vi "WLAN_FrameAnalysis.vi"(8 "error in (no error)":errorcluster, 10 "Decode SC":bool, 11 "input cluster":cluster{"t0":dbl, "dt":dbl, "Y":cdb[]}) -> (0 "error out":errorcluster, 1 "Constellation":cdb[](graph), 2 "Modulation parameter":T1, 3 "output bits":i8[](array[numeric]), 4 "Frequency offset":dbl, 5 "SIG valid?":bool, 6 "FFT":dbl[](graph))   [LabVIEW 2022 SP3]
panel:
  out "x+y":dbl
  out "Frequency offset(LTF)":dbl
  out "Frequency offset corrected signal 2":cluster{"t0":dbl, "dt":dbl, "Y":dbl[]}(graph)
  out "size(s) 3":i32
  out "size(s) 2":i32
  out "size(s)":i32
  out "Symbol numbers":i32
  out "encoded bit numbers":u32
  out "original bit numbers":u32
  out "Channel Esitimate":dbl[](graph)
  out "Frequency offset corrected signal":cluster{"t0":dbl, "dt":dbl, "Y":dbl[]}(graph)
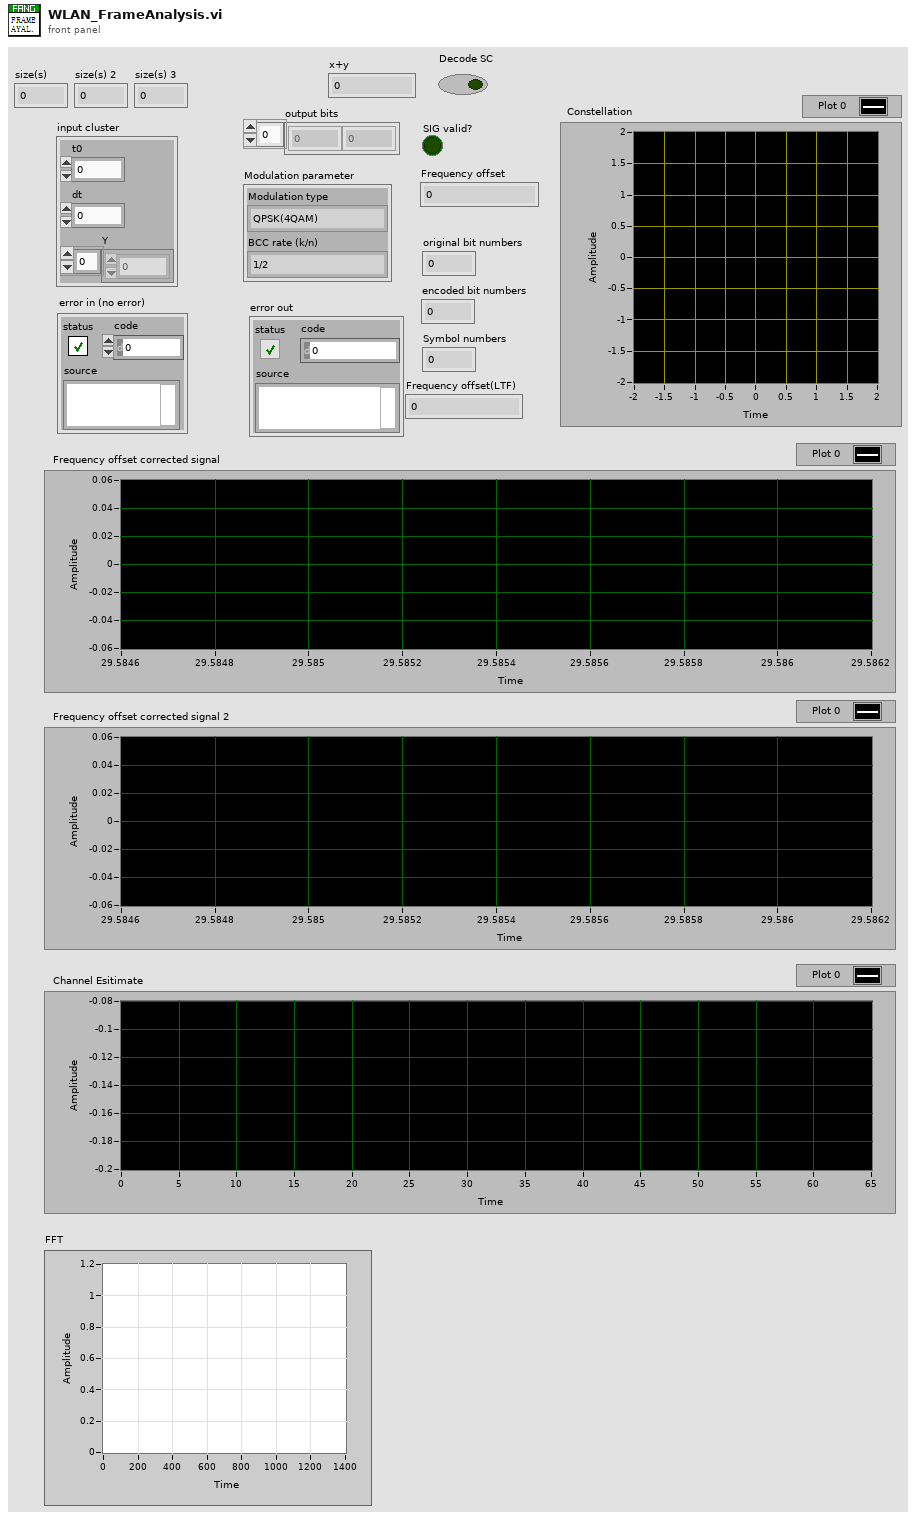
[diagram p1: front panel]
types:
  T1 = cluster{"Modulation type":enum16{"QPSK(4QAM)", "64QAM", "16QAM", "BPSK"}, "BCC rate (k/n)":enum16{"1/2", "2/3", "3/4"}}
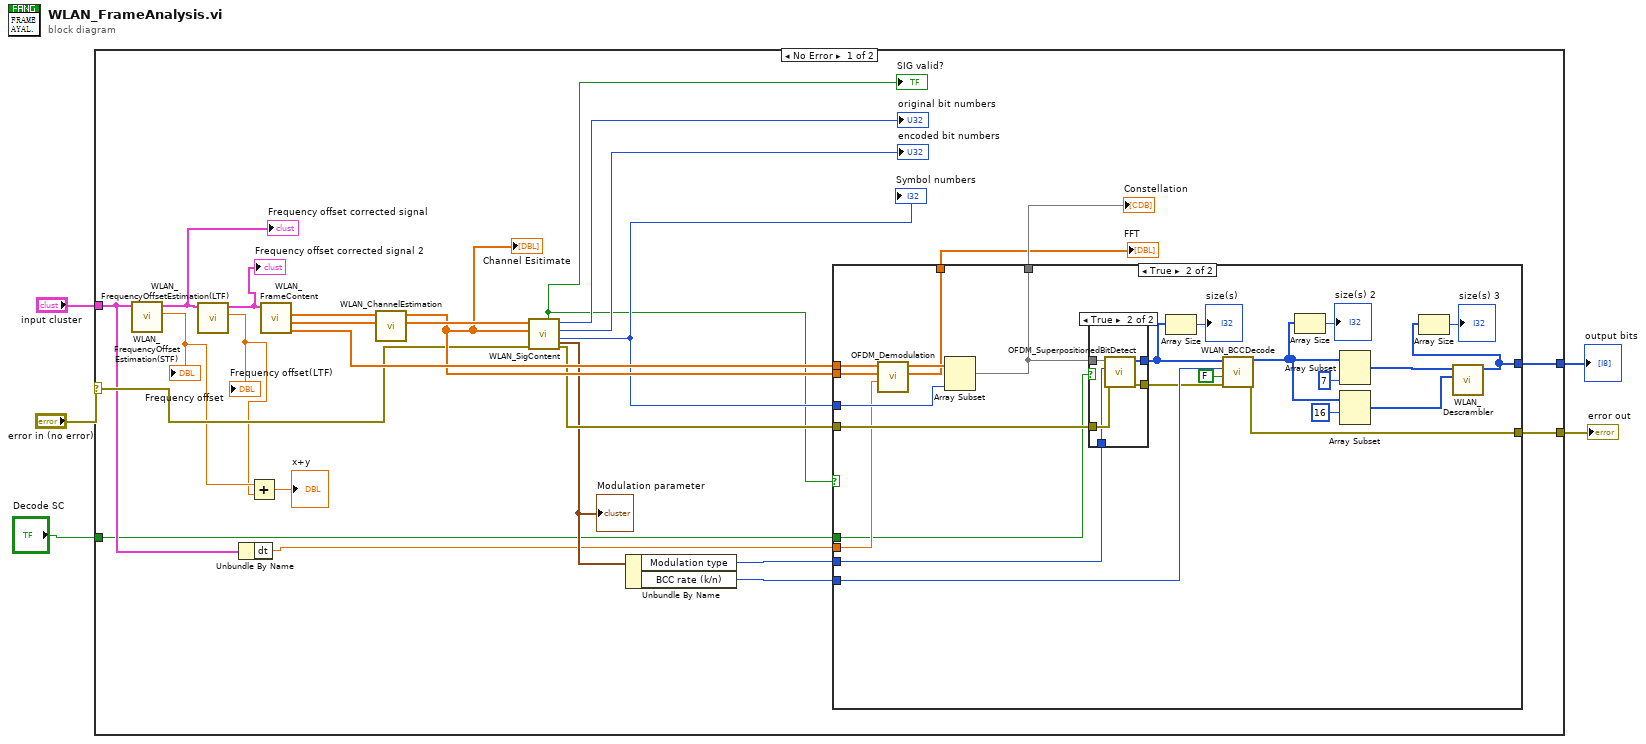
[diagram p0: block diagram]
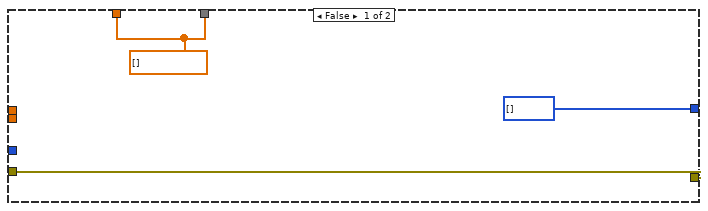
[diagram p2: hidden frame]
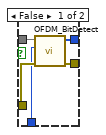
[diagram p3: hidden frame]
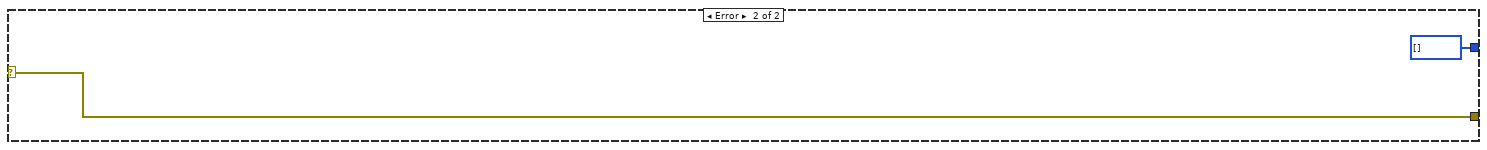
[diagram p4: hidden frame]
diagram:
  n1 = case shown="No Error" "error in (no error)" {
    selector: "error in (no error)" -> [w15 w68]
    tunnel: "input cluster" -> [w9 _]
    tunnel: [w22 w68] -> w4
    tunnel: [w21 i8[] [] ("scrambled bits")] -> w3
    tunnel: "Decode SC" -> [w7 _]
    frame No Error {
      n2 = call "WLAN_FrequencyOffsetEstimation(STF).vi"("output cluster"=w9) -> ("Frequency offset(STF)"=w13:dbl, "output cluster 2"=w14:cluster{"t0":dbl, "dt":dbl, "Y":cdb[]})  [unwired: 8 in]
      "Frequency offset corrected signal" <- w14
      "Frequency offset" <- w13
      n3 = call "WLAN_FrequencyOffsetEstimation(LTF).vi"("input cluster"=w14) -> ("Frequency offset(LTF)"=w12:dbl, "output cluster"=w10:cluster{"t0":dbl, "dt":dbl, "Y":cdb[]})  [unwired: 9 in]
      "Frequency offset corrected signal 2" <- w10
      "Frequency offset(LTF)" <- w12
      n4 = Unbundle By Name(w9) -> ("dt"=w8:dbl)
      n5 = Add(x=w13, y=w12) -> (x+y=→"x+y":dbl)
      n6 = call "WLAN_FrameContent.vi"("Input cluster"=w10) -> ("DATA"=w30:cdb[], "SIG"=w28:cdb[], "LTF"=w29:cdb[])  [unwired: 7 in, 1 out]
      n7 = call "WLAN_ChannelEstimation.vi"("LTF"=w29) -> ("Frequency estimation"=w27:cdb[])  [unwired: 10 in]
      "Channel Esitimate" <- w27
      n8 = call "WLAN_SigContent.vi"("error in (no error)"=w15, "Frequency channel estimation"=w27, "SIG"=w28) -> ("error out"=w26:errorcluster, "Symbol numbers"=w23:i32, "encoded bit numbers"=→"encoded bit numbers":u32, "original bit numbers"=→"original bit numbers":u32, "Modulation parameter"=w20:T1, "SIG valid?"=w16:bool)  [unwired: 3 in]
      "Modulation parameter" <- w20
      "Symbol numbers" <- w23
      "SIG valid?" <- w16
      n9 = Unbundle By Name(w20) -> ("Modulation type"=w19:enum16{"QPSK(4QAM)", "64QAM", "16QAM", "BPSK"}, "BCC rate (k/n)"=w18:enum16{"1/2", "2/3", "3/4"})
      n10 = case shown="True" w16 {
        tunnel: w30 -> [_ w57]
        tunnel: [w33 w49] -> w22
        tunnel: w27 -> [_ w55]
        tunnel: w26 -> [w33 w54]
        tunnel: w23 -> [_ w53]
        tunnel: w19 -> [_ w52]
        tunnel: [i8[] [] ("scrambled bits") w37] -> w21
        tunnel: w18 -> [_ w51]
        tunnel: [w31 w43] -> w17
        tunnel: w8 -> [_ w36]
        tunnel: w7 -> [_ w35]
        tunnel: [w31 w34] -> w6
        frame False {
          w31 = cdb[] []
        }
        frame True {
          n11 = call "OFDM_Demodulation.vi"("sampling period"=w36, "Frequency channel estimation"=w55, "Input sequence"=w57) -> ("FFT"=w34:dbl[], "Output sequence"=w56:cdb[])  [unwired: 7 in]
          n12 = Array Subset(array=w56, length=w53) -> (w43:cdb[])  [unwired: 1 in]
          n13 = case shown="True" w35 {
            tunnel: w54 -> [w62 w65]
            tunnel: w52 -> [w61 w64]
            tunnel: [w60 w63] -> w50
            tunnel: w43 -> [w59 w66]
            tunnel: [w58 w67] -> w42
            frame False {
              n14 = call "OFDM_BitDetect.vi"("Input symbols"=w59, "Modulation type"=w61, "error in (no error)"=w62) -> ("Output bits"=w58:i8[], "error out"=w60:errorcluster)  [unwired: 6 in]
            }
            frame True {
              n15 = call "OFDM_SuperpositionedBitDetect.vi"("Input symbols"=w66, "Modulation type"=w64, "error in (no error)"=w65) -> ("Output bits"=w67:i8[], "error out"=w63:errorcluster)  [unwired: 6 in]
            }
          }
          n16 = Array Size(array=w42) -> (size(s)=→"size(s)":i32)
          n17 = call "WLAN_BCCDecode.vi"("error in (no error)"=w50, "need add zeros?"=FALSE, "BCC rate (k/n)"=w51, "input bit stream"=w42) -> ("error out"=w49:errorcluster, "output bit stream"=w39:i8[])  [unwired: 6 in]
          n18 = Array Size(array=w39) -> (size(s)=→"size(s) 2":i32)
          n19 = Array Subset(array=w39, length=7) -> (w45:i8[])  [unwired: 1 in]
          n20 = Array Subset(array=w39, index=16) -> (w46:i8[])  [unwired: 1 in]
          n21 = call "WLAN_Descrambler.vi"("scrambler initial bits"=w45, "data bits"=w46) -> ("scrambled bits"=w37:i8[])  [unwired: 7 in]
          n22 = Array Size(array=w37) -> (size(s)=→"size(s) 3":i32)
        }
      }
      "Constellation" <- w17
      "FFT" <- w6
    }
    frame Error {
    }
  }
  "error out" <- w4
  "output bits" <- w3
